vi "clusters.vi"() -> ()   [LabVIEW 2018]
panel:
  out "array of clusters":cluster{cluster{string, i32, bool, dbl}}[](array[cluster])
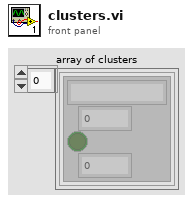
[diagram p1: front panel]
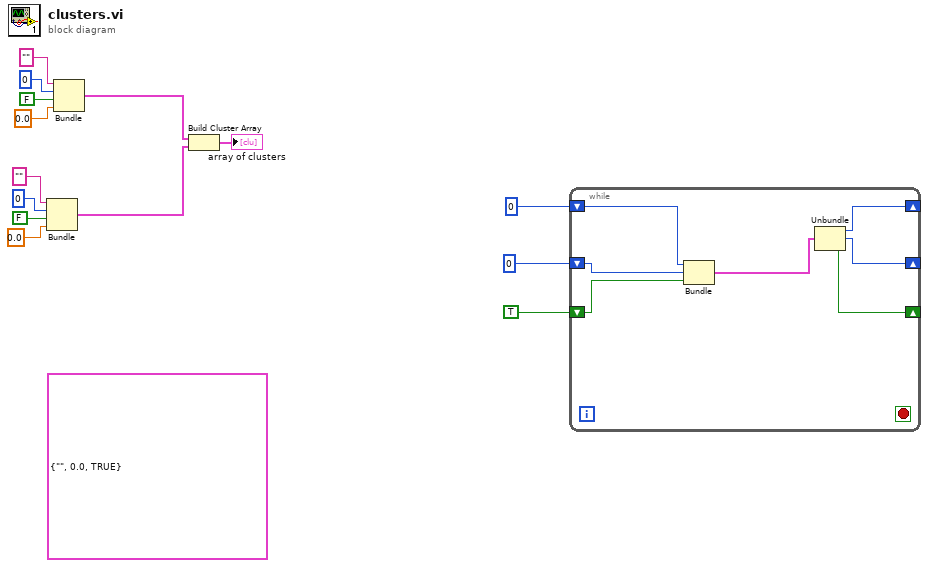
[diagram p0: block diagram]
diagram:
  (unwired) cluster{string, dbl, bool} {"", 0.0, TRUE}
  n1 = Bundle("", 0, FALSE, 0.0) -> (w5:cluster{string, i32, bool, dbl})  [unwired: 1 in]
  n2 = Bundle("", 0, FALSE, 0.0) -> (w6:cluster{string, i32, bool, dbl})  [unwired: 1 in]
  n3 = Build Cluster Array(w6, w5) -> (→"array of clusters":cluster{cluster{string, i32, bool, dbl}}[])
  n4 = while {
    shift-right: [w17] -> _
    shift-left: 0 -> [w19]
    shift-right: [w16] -> _
    shift-left: 0 -> [w20]
    shift-right: [w15] -> _
    shift-left: TRUE -> [w21]
    stop <- _ stop-if-true
    n5 = Bundle(w19, w20, w21) -> (w18:cluster{i32, i32, bool})  [unwired: 1 in]
    n6 = Unbundle(w18) -> (w17:i32, w16:i32, w15:bool)
  }
